vi "Split Namespace.vi"(7 "Separator (dot)":string, 10 "Namespaced String":string) -> (2 "String":string, 3 "Namespace":string)   [LabVIEW 2013, in "OpenConvert.lvlib"]
uses:
  OpenConvert.lvlib
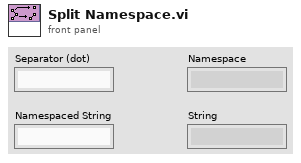
[diagram p1: front panel]
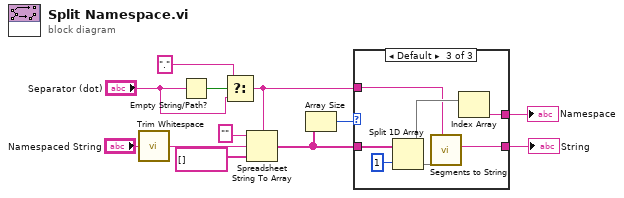
[diagram p0: block diagram]
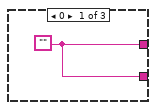
[diagram p2: hidden frame]
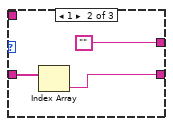
[diagram p3: hidden frame]
diagram:
  n1 = call <vilib>:"Trim Whitespace.vi"("string"="Namespaced String") -> ("trimmed string"=w12:string)  [unwired: 1 in]
  n2 = Empty String/Path?(string/path="Separator (dot)") -> (empty?=w10:bool)
  n3 = Select(t="." ("delimiter (Tab)"), s=w10, f="Separator (dot)") -> (s? t:f=w1:string)
  n4 = Spreadsheet String To Array(delimiter (Tab)=w1, format string="", spreadsheet string=w12, array type (2D Dbl)=string[] [] ("array")) -> (array=w4:string[])
  n5 = Array Size(array=w4) -> (size(s)=w5:i32)
  n6 = case shown="Default" w5 {
    tunnel: w4 -> [_ w16 w23]
    tunnel: [w13 w15 w18] -> w3
    tunnel: [w13 "" w20] -> w2
    tunnel: w1 -> [_ _ w17]
    frame 0 {
      w13 = ""
    }
    frame 1 {
      n7 = Index Array(array=w16) -> (element=w15:string)  [unwired: 1 in]
    }
    frame Default {
      n8 = Split 1D Array(array=w23, index=1) -> (first subarray=w21:string[], second subarray=w19:string[])
      n9 = call "Segments to String.vi"("Separator (dot)"=w17, "Segments"=w19) -> ("String"=w18:string)  [unwired: 9 in]
      n10 = Index Array(array=w21) -> (element=w20:string)  [unwired: 1 in]
    }
  }
  "String" <- w3
  "Namespace" <- w2
